vi "armsim-battery-simulation-exec.vi"(10 "Numeric":dbl, 11 "Motor Current":dbl) -> (3 "Voltage":dbl)   [LabVIEW 2019]
uses:
  <vilib>/Rock Robotics/WPI/ThirdParty/JAS_Junk/TrajLib/Trajectory_Library.lvlib
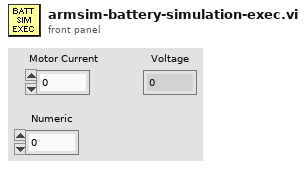
[diagram p1: front panel]
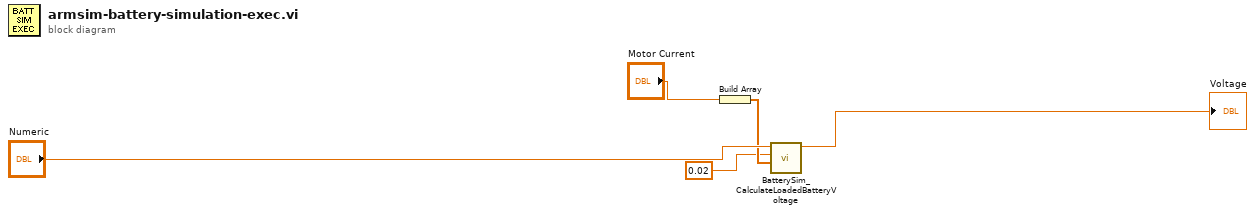
[diagram p0: block diagram]
diagram:
  n1 = Build Array("Motor Current") -> (w2:dbl[])
  n2 = call <vilib>:"BatterySim_CalculateLoadedBatteryVoltage.vi"("Currents"=w2, "Resistance_Ohms"=0.02, "NominalVoltage"="Numeric") -> ("Voltage"=→"Voltage":dbl)  [unwired: 8 in]
